vi "FakeTheory.vi"(10 "Input Data":string) -> (0 "error out":errorcluster)   [LabVIEW 2019, in "TestCaseTestSupport.lvlib"]
uses:
  TestCaseTestSupport.lvlib
  Assertion/Assertion.lvlib
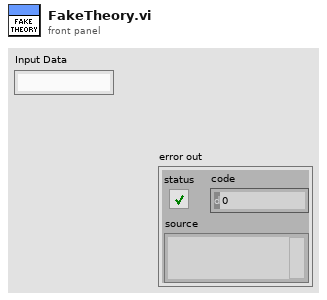
[diagram p1: front panel]
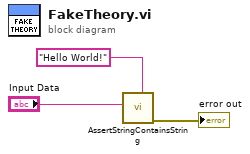
[diagram p0: block diagram]
diagram:
  n1 = call "AssertStringContainsString.vi"("Needle"="Hello World!", "Haystack"="Input Data") -> ("error out"=→"error out":errorcluster)  [unwired: 9 in]
